vi "Read.vi"(8 "error in (no error)":errorcluster, 11 "DAQmx DIO in":refnum<class "DAQmx DIO.lvclass">) -> (0 "error out":errorcluster, 2 "Output":variant, 3 "DAQmx DIO out":refnum<class "DAQmx DIO.lvclass">)   [LabVIEW 2017, in "DAQmx DIO.lvclass"]
uses:
  DAQmx DIO.lvclass
  DAQmx/DAQmx.lvclass
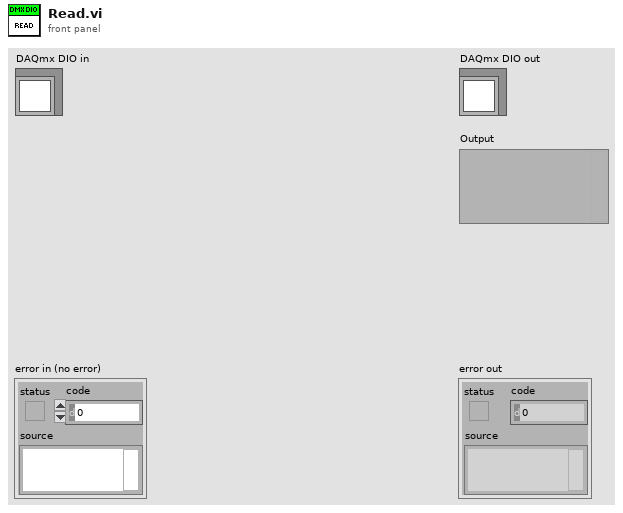
[diagram p1: front panel]
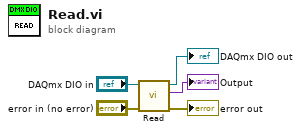
[diagram p0: block diagram]
diagram:
  n1 = call-parent "Read.vi"("error in (no error)"="error in (no error)", "DAQmx in"="DAQmx DIO in") -> ("error out"=→"error out":errorcluster, "Output"=→"Output":variant, "DAQmx out"=→"DAQmx DIO out":refnum<class "DAQmx DIO.lvclass">)  [unwired: 7 in]
